vi "scriptnode.vi"   [LabVIEW 2014]
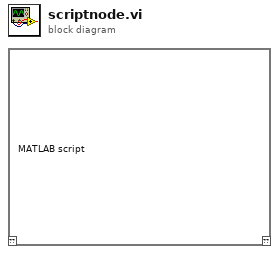
[diagram p0: block diagram]
diagram:
  n1 = script code="MATLAB script"() -> ()  [unwired: 1 in, 1 out]
